vi "ORS_AlazarDLLAcq_XferLatestFrame.vi"(9 "FrameNumToDisplay":i32=1, 10 "SamplesPerBuffer":u32, 11 "ATSHandle":u32[](array[numeric])) -> (1 "Return Code":u32=589, 2 "Buffer":u16[](array[numeric]), 3 "ATSHandleOut":u32=60940)   [LabVIEW 2021]
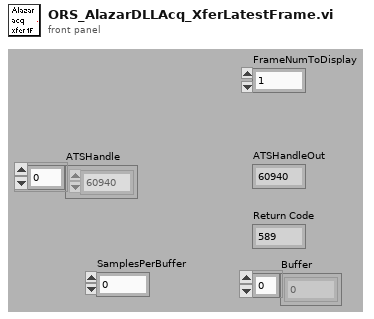
[diagram p1: front panel]
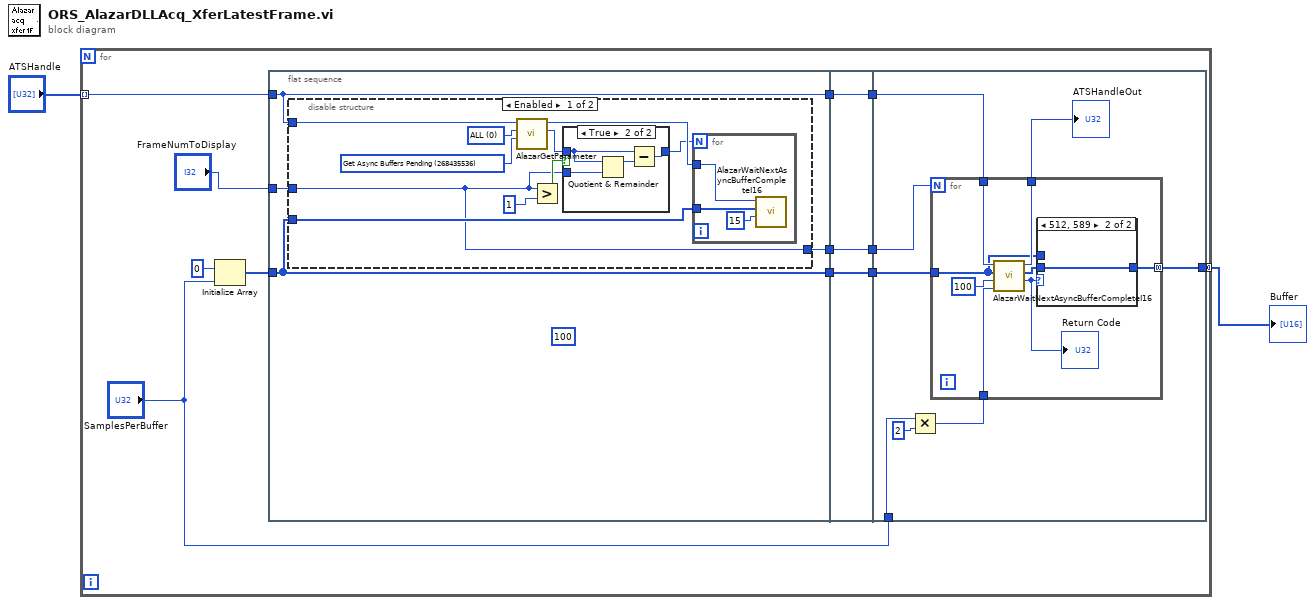
[diagram p0: block diagram]
diagram:
  n1 = for {
    tunnel: [w11] -> w2 mode=concatenating
    tunnel: "ATSHandle" -> [w10] mode=indexing
    n2 = Initialize Array(i16 0 ("element"), "SamplesPerBuffer") -> (w12:i16[])
    n3 = flat-sequence {
      tunnel: w10 -> [w17]
      tunnel: w12 -> [w18]
      tunnel: [w18] -> w8
      tunnel: [w17] -> w6
      tunnel: "FrameNumToDisplay" -> [w16]
      tunnel: [w15] -> w4
      tunnel: w8 -> [w40]
      tunnel: [w40] -> w7
      tunnel: w6 -> [w39]
      tunnel: [w39] -> w5
      tunnel: w4 -> [w38]
      tunnel: [w38] -> w3
      tunnel: "SamplesPerBuffer" -> [w44]
      tunnel: w7 -> [w43]
      tunnel: [w42] -> w11
      tunnel: w5 -> [w48]
      tunnel: w3 -> [w41]
      frame #0 {
        (unwired) 100 ("Numeric")
        n4 = disable-structure shown="Enabled" {
          disable-tunnel: w18 -> [w28 _]
          disable-tunnel: w17 -> [w27 _]
          disable-tunnel: w16 -> [w20 w37]
          disable-tunnel: [w20 w37] -> w15
          frame Enabled {
            w24 = u32 268435536 items=["Data Width"=268435465, "Set/Get Async BuffSize"=268435513, "Set/Get Async Buffcount"=268435520, "Get Data Format"=268435522, "Get Samples Per Timestamp Clock"=268435524, "Get Records Captured"=268435525, "Get Async Buffers Pending"=268435536, "Get Async Buffers Pending Full"=268435537, "Get Async Buffers Pending Empty"=268435538, "ECC Mode"=268435528, "Get Aux Input Level"=268435529, "Get Channels Per Board"=268435568, "Pack Mode"=268435570, "Get FPGA Temperature"=268435584] ("Parameter")
            w25 = u8 0 items=["ALL"=0, "A"=1, "B"=2, "C"=4, "D"=8] ("Channel")
            n5 = call "AlazarGetParameter.vi"("Parameter"=w24, "Channel"=w25, "Handle"=w27) -> ("Value"=w23:i32, "Handle"=w26:u32)  [unwired: 1 in, 2 out]
            n6 = Greater?(x=w20, y=1) -> (0:w21:bool)
            n7 = case shown="True" w21 {
              tunnel: w23 -> [w29 w33]
              tunnel: [w29 w32] -> w19
              tunnel: w20 -> [_ w30]
              frame False {
              }
              frame True {
                n8 = Quotient & Remainder(x=w33, y=w30) -> (x-y*floor(x/y)=w31:i32)  [unwired: 1 out]
                n9 = Subtract(x=w33, y=w31) -> (x-y=w32:i32)
              }
            }
            n10 = for {
              N: w19 -> [_]
              tunnel: w28 -> [w36]
              tunnel: w26 -> [w35]
              n11 = call "AlazarWaitNextAsyncBufferCompleteI16.vi"("timeout_ms"=u32 15, "Buffer"=w36, "Handle"=w35) -> ()  [unwired: 2 in, 3 out]
            }
          }
          frame Disabled {
          }
        }
      }
      frame #1 {
      }
      frame #2 {
        n12 = Multiply(x=w44, y=u32 2) -> (x*y=w45:u32)
        n13 = for {
          N: w41 -> [_]
          tunnel: w48 -> [w56]
          tunnel: [w55] -> w47
          tunnel: w45 -> [w51]
          tunnel: w43 -> [w50]
          tunnel: [w49] -> w42 mode=concatenating
          n14 = call "AlazarWaitNextAsyncBufferCompleteI16.vi"("bytesToCopy"=w51, "timeout_ms"=u32 100, "Buffer"=w50, "Handle"=w56) -> ("Return Code"=w52:u32, "Buffer"=w53:u16[], "Handle"=w55:u32)  [unwired: 1 in]
          "Return Code" <- w52
          n15 = case shown="512, 589" w52 {
            tunnel: w50 -> [w57 _]
            tunnel: [w57 w58] -> w49
            tunnel: w53 -> [_ w58]
            frame 0, Default {
            }
            frame 512, 589 {
            }
          }
        }
        "ATSHandleOut" <- w47
      }
    }
  }
  "Buffer" <- w2
